vi "AFM_Driver_Manager.InsertActiveIntoSubpanel.vi"(8 "error in (no error)":errorcluster, 10 "SubPnl Refnum":refnum<vi>, 11 "AFM_Driver_Manager in":refnum<class "AFM_Driver_Manager.lvclass">) -> (0 "error out":errorcluster, 3 "AFM_Driver_Manager out":refnum<class "AFM_Driver_Manager.lvclass">)   [LabVIEW 2019, in "AFM_Driver_Manager.lvclass"]
uses:
  AFM_Driver_Manager.lvclass
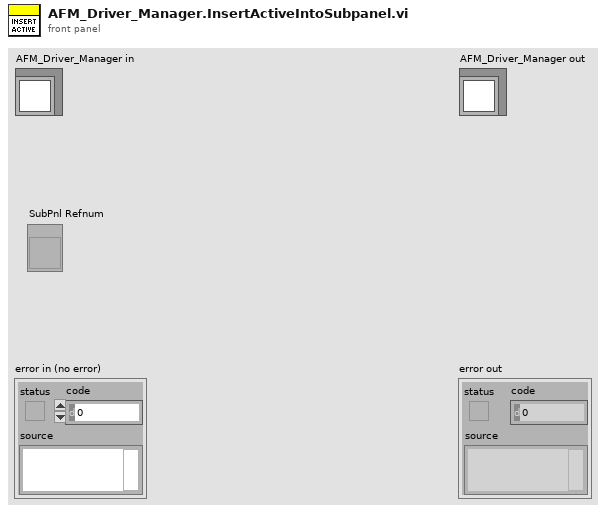
[diagram p1: front panel]
types:
  T1 = typedef "AFM_Driver_Manager.lvclass/AFM_Driver_Manager.PublicMethods.ctl" = cluster{"Stop Event":refnum<user-event>, "Lithography Data":refnum<user-event>, "Run Lithography":refnum<user-event>, "Background Image":refnum<user-event>, "Abort Notifier":refnum<user-event>}
  T2 = cluster{"VI Refnum":refnum<vi>, "Path":path, "Name":string, "Events":T1}
  T3 = enum32{"Invalid", "Standard", "Closed", "Hidden", "Minimized", "Maximized"}
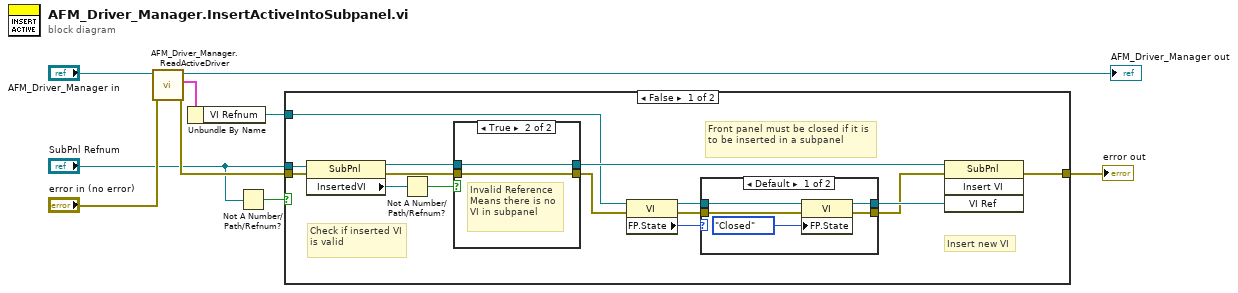
[diagram p0: block diagram]
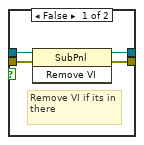
[diagram p3: hidden frame]
diagram:
  n1 = call "AFM_Driver_Manager.ReadActiveDriver.vi"("error in (no error)"="error in (no error)", "AFM_Driver_Manager in"="AFM_Driver_Manager in") -> ("error out"=w7:errorcluster, "Active Driver"=w2:T2, "AFM_Driver_Manager out"=→"AFM_Driver_Manager out":refnum<class "AFM_Driver_Manager.lvclass">)  [unwired: 7 in]
  n2 = Unbundle By Name(w2) -> ("VI Refnum"=w1:refnum<vi>)
  n3 = Not A Number/Path/Refnum?(number/path/refnum="SubPnl Refnum") -> (NaN/Path/Refnum?=w3:bool)
  n4 = case shown="False" w3 {
    tunnel: "SubPnl Refnum" -> [w20 _]
    tunnel: w1 -> [w16 _]
    tunnel: w7 -> [w23 w38]
    tunnel: [w22 w38] -> w8
    frame False {
      # "Front panel must be closed if it is to be inserted in a subpanel"
      # "Insert new VI"
      # "Check if inserted VI is valid"
      n5 = property class="SubPnl"(reference=w20, error in=w23) -> (reference out=w18:refnum<vi>, error out=w24:errorcluster, "InsertedVI"=w21:refnum<vi>)
      n6 = Not A Number/Path/Refnum?(number/path/refnum=w21) -> (NaN/Path/Refnum?=w19:bool)
      n7 = case shown="True" w19 {
        tunnel: w18 -> [w33 w36]
        tunnel: [w32 w36] -> w17
        tunnel: [w34 w37] -> w11
        tunnel: w24 -> [w35 w37]
        frame False {
          # "Remove VI if its in there"
          n8 = invoke class="SubPnl" method="Remove VI"(reference=w33, error in=w35) -> (reference out=w32:refnum<vi>, error out=w34:errorcluster)  [unwired: 1 in, 1 out]
        }
        frame True {
          # "Invalid Reference\nMeans there is no VI in subpanel"
        }
      }
      n9 = property class="VI"(reference=w16, error in=w11) -> (reference out=w15:refnum<vi>, error out=w14:errorcluster, "FP.State"=w13:T3)
      n10 = case shown="Default" w13 {
        tunnel: w15 -> [w29 w30]
        tunnel: [w26 w31] -> w10
        tunnel: w14 -> [w28 w31]
        tunnel: [w25 w30] -> w12
        frame Default {
          n11 = property class="VI"(reference=w29, error in=w28, "FP.State"=T3."Closed" ("Front Panel Window:State")) -> (reference out=w25:refnum<vi>, error out=w26:errorcluster)
        }
        frame "Closed" {
        }
      }
      n12 = invoke class="SubPnl" method="Insert VI"(reference=w17, error in=w10, "VI Ref"=w12) -> (error out=w22:errorcluster)  [unwired: 1 in, 3 out]
    }
    frame True {
      # "Subpanel Reference is invalid. Dont do anything"
    }
  }
  "error out" <- w8
